vi "Get SLSC Switch Description.vi"(8 "error in":errorcluster, 11 "slsc switch custom device in":T1 format="%.0x") -> (0 "error out":errorcluster, 2 "description":string, 3 "slsc switch custom device out":T1 format="%.0x")   [LabVIEW 2020, in "SLSC Switch Scripting.lvlib"]
doc: "Returns the description for the SLSC Switch custom device."
uses:
  SLSC Switch Scripting.lvlib
  <vilib>/NI VeriStand/Custom Device API/Custom Device Item Ref.ctl
  <vilib>/NI VeriStand/Custom Device API/Custom Device API.lvlib
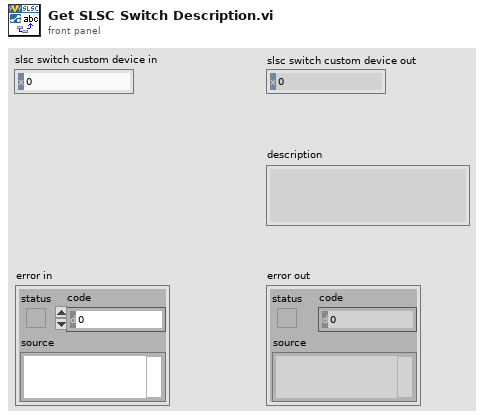
[diagram p1: front panel]
types:
  T1 = typedef "Custom Device API.lvlib/Custom Device Item Ref.ctl" = u64
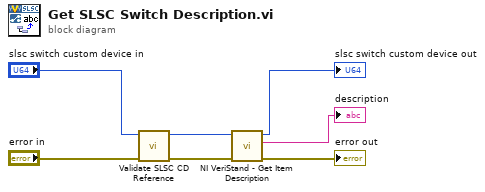
[diagram p0: block diagram]
diagram:
  n1 = call "Validate SLSC CD Reference.vi"("error in"="error in", "slsc switch custom device in"="slsc switch custom device in") -> ("error out"=w3:errorcluster, "slsc switch custom device out"=w1:T1)  [unwired: 8 in]
  n2 = call <vilib>:"NI VeriStand - Get Item Description.vi"("error in (no error)"=w3, "Item Ref in"=w1) -> ("error out"=→"error out":errorcluster, "Description"=→"description":string, "Item Ref out"=→"slsc switch custom device out":T1)  [unwired: 6 in, 1 out]
